vi "test_Add_Conpane.vi"() -> ()   [LabVIEW 2015]
uses:
  <vilib>/Utility/miscctls.llb/LVRectTypeDef.ctl
panel:
  in  "F":dbl
  in  "E":dbl
  in  "D":dbl
  in  "B":dbl
  in  "A":dbl
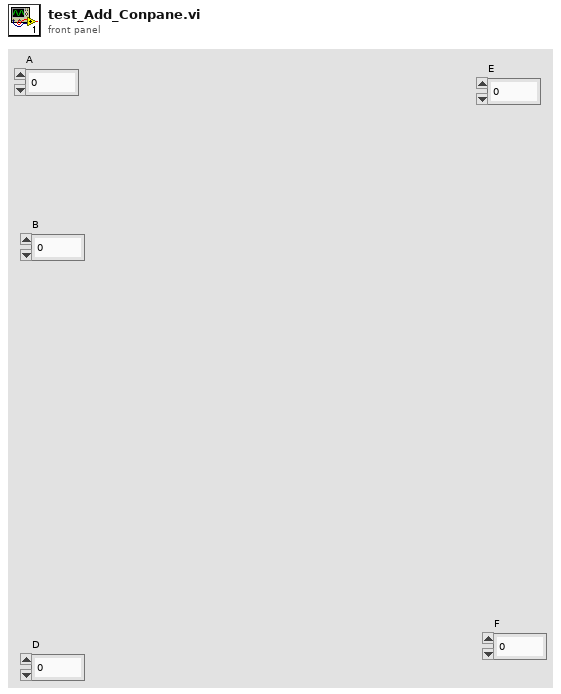
[diagram p1: front panel]
types:
  T1 = typedef "LVRectTypeDef.ctl" = cluster{"Left":i16, "Top":i16, "Right":i16, "Bottom":i16}
  T2 = typedef "LVPositionTypeDef.ctl" = cluster{"Left":i32, "Top":i32}
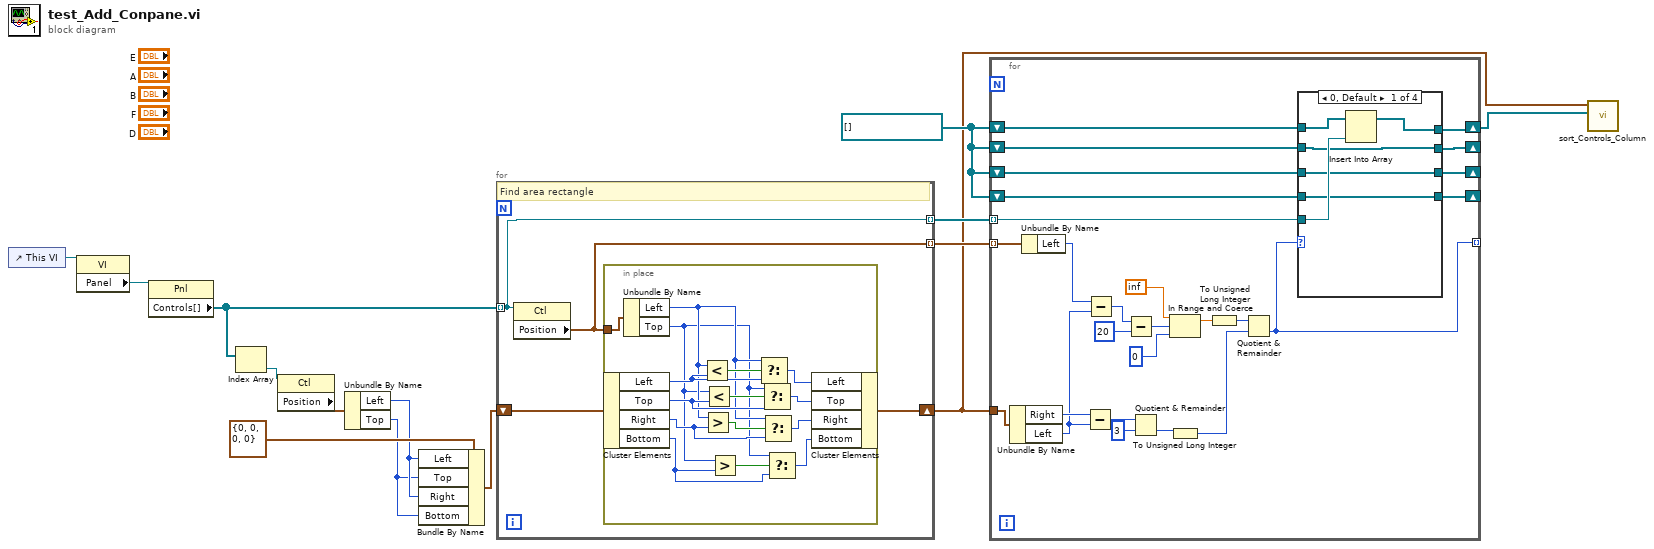
[diagram p0: block diagram]
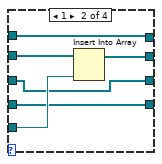
[diagram p2: hidden frame]
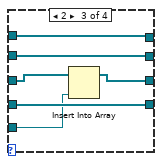
[diagram p3: hidden frame]
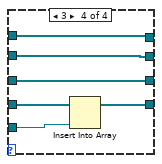
[diagram p4: hidden frame]
diagram:
  w3 = refnum<vi>[] []
  n1 = control-ref of="This VI"() -> (w14:refnum<vi>)
  n2 = property class="VI"(reference=w14) -> ("Panel"=w13:refnum<vi>)  [unwired: 1 in, 2 out]
  n3 = property class="Pnl"(reference=w13) -> ("Controls[]"=w10:refnum<vi>[])  [unwired: 1 in, 2 out]
  n4 = Index Array(array=w10) -> (element=w9:refnum<vi>)  [unwired: 1 in]
  n5 = property class="Ctl"(reference=w9) -> ("Position"=w6:T2)  [unwired: 1 in, 2 out]
  n6 = Unbundle By Name(w6) -> ("Left"=w5:i32, "Top"=w4:i32)
  n7 = Bundle By Name(cluster=T1 {"Left"=0, "Top"=0, "Right"=0, "Bottom"=0} ("Master Bounds Rect"), "Left"=w5, "Top"=w4, "Right"=w5, "Bottom"=w4) -> (w7:T1)
  n8 = for {
    tunnel: w10 -> [w15] mode=indexing
    shift-right: [w17] -> w1
    shift-left: w7 -> [w18]
    tunnel: [w16] -> w11 mode=indexing
    tunnel: [w15] -> w12 mode=indexing
    # "Find area rectangle"
    n9 = property class="Ctl"(reference=w15) -> ("Position"=w16:T2)  [unwired: 1 in, 2 out]
    n10 = in-place {
      in-place-border: w16 -> [w33]
      n11 = in-place-cluster #1(w18) -> ("Left"=w32:i16, "Top"=w28:i16, "Right"=w26:i16, "Bottom"=w20:i16)
      n12 = Unbundle By Name(w33) -> ("Left"=w27:i32, "Top"=w21:i32)
      n13 = Less?(x=w27, y=w32) -> (x < y?=w30:bool)
      n14 = Greater?(x=w27, y=w26) -> (0:w23:bool)
      n15 = Less?(x=w21, y=w28) -> (x < y?=w29:bool)
      n16 = Greater?(x=w21, y=w20) -> (0:w22:bool)
      n17 = Select(t=w27, s=w30, f=w32) -> (s? t:f=w31:i32)
      n18 = Select(t=w21, s=w29, f=w28) -> (s? t:f=w24:i32)
      n19 = Select(t=w27, s=w23, f=w26) -> (s? t:f=w25:i32)
      n20 = Select(t=w21, s=w22, f=w20) -> (s? t:f=w19:i32)
      n21 = in-place-cluster #1("Left"=w31, "Top"=w24, "Right"=w25, "Bottom"=w19) -> (w17:T1)
    }
  }
  n22 = for {
    tunnel: w12 -> [w38] mode=indexing
    tunnel: w11 -> [w55] mode=indexing
    tunnel: w1 -> [w59]
    tunnel: [w43] -> _ mode=indexing
    shift-right: [w37] -> w2
    shift-left: w3 -> [w42]
    shift-right: [w36] -> _
    shift-left: w3 -> [w41]
    shift-right: [w35] -> _
    shift-left: w3 -> [w40]
    shift-right: [w34] -> _
    shift-left: w3 -> [w39]
    n23 = Unbundle By Name(w59) -> ("Right"=w58:i16, "Left"=w53:i16)
    n24 = Unbundle By Name(w55) -> ("Left"=w54:i32)
    n25 = Subtract(x=w58, y=w53) -> (x-y=w57:i16)
    n26 = Subtract(x=w54, y=w53) -> (x-y=w52:i32)
    n27 = Subtract(x=w52, y=20) -> (x-y=w48:i32)
    n28 = Quotient & Remainder(x=w57, y=i16 3) -> (floor(x/y)=w50:i16)  [unwired: 1 out]
    n29 = In Range and Coerce(upper limit=inf, x=w48, lower limit=0) -> (coerced(x)=w45:dbl)  [unwired: 1 out]
    n30 = To Unsigned Long Integer(number=w50) -> (unsigned 32bit integer=w49:u32)
    n31 = To Unsigned Long Integer(number=w45) -> (unsigned 32bit integer=w44:u32)
    n32 = Quotient & Remainder(x=w44, y=w49) -> (floor(x/y)=w43:u32)  [unwired: 1 out]
    n33 = case shown="0, Default" w43 {
      tunnel: w42 -> [w65 w68 w77 w83]
      tunnel: w41 -> [w62 w71 w75 w79]
      tunnel: w40 -> [w61 w67 w74 w78]
      tunnel: w39 -> [w60 w66 w76 w82]
      tunnel: w38 -> [w64 w70 w72 w80]
      tunnel: [w63 w68 w77 w83] -> w37
      tunnel: [w62 w69 w75 w79] -> w36
      tunnel: [w61 w67 w73 w78] -> w35
      tunnel: [w60 w66 w76 w81] -> w34
      frame 0, Default {
        n34 = Insert Into Array(array=w65, new element=w64) -> (w63:refnum<vi>[])  [unwired: 1 in]
      }
      frame 1 {
        n35 = Insert Into Array(array=w71, new element=w70) -> (w69:refnum<vi>[])  [unwired: 1 in]
      }
      frame 2 {
        n36 = Insert Into Array(array=w74, new element=w72) -> (w73:refnum<vi>[])  [unwired: 1 in]
      }
      frame 3 {
        n37 = Insert Into Array(array=w82, new element=w80) -> (w81:refnum<vi>[])  [unwired: 1 in]
      }
    }
  }
  n38 = call "sort_Controls_Column.vi"("Controls"=w2, "Area Scale"=w1) -> ()  [unwired: 10 in]
